vi "Read Active Channel.vi"(8 "error in (no error)":errorcluster, 11 "FunctionGenerator in":refnum<class "FunctionGenerator.lvclass">) -> (0 "error out":errorcluster, 2 "Active Channel":i32, 3 "FunctionGenerator out":refnum<class "FunctionGenerator.lvclass">)   [LabVIEW 2019, in "FunctionGenerator.lvlib" / "FunctionGenerator.lvclass"]
uses:
  Library/FunctionGenerator.lvclass
  Library/FunctionGenerator.lvclass/FunctionGenerator.ctl
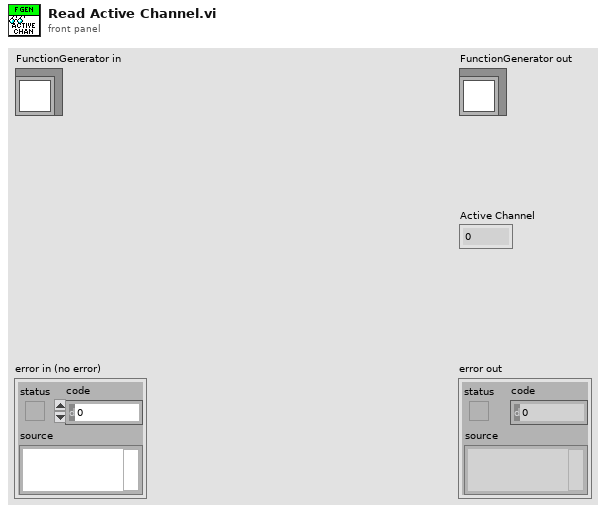
[diagram p1: front panel]
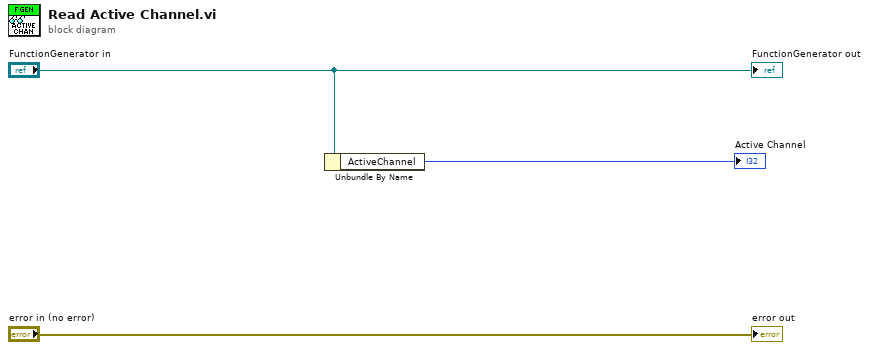
[diagram p0: block diagram]
diagram:
  n1 = Unbundle By Name("FunctionGenerator in") -> ("ActiveChannel"=→"Active Channel":i32)
  "error out" <- "error in (no error)"
  "FunctionGenerator out" <- "FunctionGenerator in"
